vi "Vector3_Cross_Product.vi"(1 "V":dbl[](array[numeric])=[0.0, 1.0, 0.0], 2 "U":dbl[](array[numeric])=[1.0, 0.0, 0.0]) -> (0 "UxV":dbl[](array[numeric])=[0.0, 0.0, 1.0])   [LabVIEW 2010]
panel:
  # "Finds vector perpendicular to U and V (Right handed)"
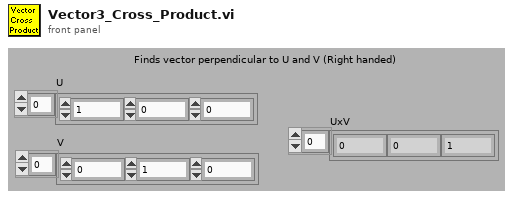
[diagram p1: front panel]
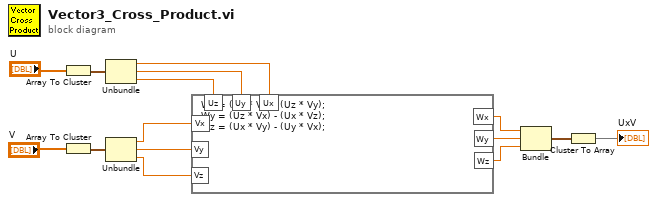
[diagram p0: block diagram]
diagram:
  n1 = Array To Cluster(array="U") -> (cluster=w14:cluster{"U[0]":dbl, "U[1]":dbl, "U[2]":dbl})
  n2 = Array To Cluster(array="V") -> (cluster=w13:cluster{"V[0]":dbl, "V[1]":dbl, "V[2]":dbl})
  n3 = Unbundle(w14) -> ("U[0]"=w6:dbl, "U[1]"=w5:dbl, "U[2]"=w4:dbl)
  n4 = Unbundle(w13) -> ("V[0]"=w3:dbl, "V[1]"=w2:dbl, "V[2]"=w1:dbl)
  n5 = formula code="Wx = (Uy * Vz) - (Uz * Vy);\nWy = (Uz * Vx) - (Ux * Vz);\nWz = (Ux * Vy) - (Uy * Vx);"("Ux"=w6, "Uy"=w5, "Uz"=w4, "Vx"=w3, "Vy"=w2, "Vz"=w1) -> ("Wx"=w11:dbl, "Wy"=w10:dbl, "Wz"=w9:dbl)
  n6 = Bundle("Wx"=w11, "Wy"=w10, "Wz"=w9) -> (w8:cluster{"Wx":dbl, "Wy":dbl, "Wz":dbl})  [unwired: 1 out]
  n7 = Cluster To Array(cluster=w8) -> (array=→"UxV":dbl[])
